vi "Lab Panel V5.10.vi"() -> ()   [LabVIEW 2013] (continued)
                            n1484 = TDMS Write(0:w2790, 5:"TEST PASS", 7:w2794, 9:w2793) -> (15:w2796:errorcluster)  [unwired: 2 in, 3 out]
                            n1485 = local write "data file error"(w2796) -> ()
                          }
                          frame #1 {
                            n1486 = Bundle(cluster=w2797, "STATUS"="T-RISE PASS") -> (w2799:T4)  [unwired: 2 in]
                            n1487 = local write "RESULT LAB05-2"(TRUE) -> ()
                            n1488 = local write "DISP LAB05-2"(w2799) -> ()
                          }
                        }
                      }
                      frame False {
                      }
                    }
                  }
                }
              }
            }
          }
          frame #6 {
            # "end test & close test files"
            n1489 = local read "MAIL SETTINGS"() -> (w2805:T7)
            n1490 = Unbundle(w2805) -> ("OUT SERVER ADDRESS"=w2804:string, "FROM ACCOUNT"=w2803:string)  [unwired: 5 out]
            n1491 = stacked-sequence {
              tunnel: w2815 -> [_ _ _ _ _ _ _ _ _ _]
              tunnel: w2816 -> [_ _ _ _ _ _ _ _ _ _]
              tunnel: w2814 -> [_ _ _ _ _ _ _ _ _ _]
              tunnel: w2813 -> [_ _ _ _ _ _ _ _ _ _]
              tunnel: w2812 -> [_ _ _ _ _ _ _ _ _ _]
              tunnel: w2811 -> [_ _ _ _ _ _ _ _ _ _]
              tunnel: w2810 -> [_ _ _ _ _ _ _ _ _ _]
              tunnel: w2809 -> [_ _ _ _ _ _ _ _ _ _]
              tunnel: w2808 -> [_ _ _ _ _ _ _ _ _ _]
              tunnel: w2807 -> [_ _ _ _ _ _ _ _ _ _]
              tunnel: w2804 -> [w2820 w2872 w2920 w2967 w3014 w3061 w3108 w3155 w3202 w3249]
              tunnel: w2803 -> [w2819 w2871 w2919 w2966 w3013 w3060 w3107 w3154 w3201 w3248]
              tunnel: "Mail Test File To:" -> [w2818 w2870 w2918 w2965 w3012 w3059 w3106 w3153 w3200 w3247]
              tunnel: "Mail Test Fail" -> [w2817 w2869 w2917 w2964 w3011 w3058 w3105 w3152 w3199 w3246]
              frame #0 {
                # "LAB01-1"
                n1492 = local read "DISP LAB01-1"() -> (w2824:T4)
                n1493 = local read "run lab01-1"() -> (w2821:bool)
                n1494 = local read "TDMS LAB01-1"() -> (w2822:refnum<k34>)
                n1495 = Unbundle(w2824) -> ("CYCLE"=w2825:dbl, "STATUS"=w2823:string)  [unwired: 1 out]
                n1496 = case shown="True" w2821 {
                  tunnel: w2825 -> [_ w2831]
                  tunnel: w2824 -> [_ w2833]
                  tunnel: w2823 -> [_ w2830]
                  tunnel: w2822 -> [_ w2832]
                  tunnel: w2820 -> [_ w2829]
                  tunnel: w2819 -> [_ w2828]
                  tunnel: w2818 -> [_ w2827]
                  tunnel: w2817 -> [_ w2826]
                  frame False {
                  }
                  frame True {
                    n1497 = Not Equal?(x=w2830, y="RUN") -> (x != y?=w2834:bool)
                    n1498 = Greater?(x=w2831, y=2.0) -> (0:w2836:bool)
                    n1499 = And(x=w2836, y=w2834) -> (x .and. y?=w2835:bool)
                    n1500 = case shown="True" w2835 {
                      tunnel: w2833 -> [_ w2846]
                      tunnel: w2832 -> [_ w2845]
                      tunnel: w2831 -> [_ w2844]
                      tunnel: w2830 -> [_ w2843]
                      tunnel: w2829 -> [_ w2842]
                      tunnel: w2828 -> [_ w2841]
                      tunnel: w2827 -> [_ w2840]
                      tunnel: w2826 -> [_ w2839]
                      frame False {
                      }
                      frame True {
                        n1501 = stacked-sequence {
                          tunnel: w2846 -> [w2850 _ _]
                          tunnel: w2845 -> [_ w2852 _]
                          tunnel: w2844 -> [_ _ _]
                          tunnel: w2843 -> [_ _ w2858]
                          tunnel: w2842 -> [_ _ w2857]
                          tunnel: w2841 -> [_ _ w2856]
                          tunnel: w2840 -> [_ _ w2855]
                          tunnel: w2839 -> [_ _ w2854]
                          frame #0 {
                            w2847 = FALSE
                            n1502 = local write "mail control"("END") -> ()
                            n1503 = Bundle(cluster=w2850) -> (w2849:T4)  [unwired: 3 in]
                            n1504 = local write "DISP LAB01-1"(w2849) -> ()
                            n1505 = local write "O/I  LAB01-1"(w2847) -> ()
                            n1506 = local write "run lab01-1"(w2847) -> ()
                            n1507 = local write "RUN LAB01-1"(w2847) -> ()
                          }
                          frame #1 {
                            n1508 = TDMS Close(11:w2852) -> (0:w2851:errorcluster)  [unwired: 1 in, 1 out]
                            n1509 = local write "data file error"(w2851) -> ()
                          }
                          frame #2 {
                            n1510 = stacked-sequence {
                              tunnel: "LAB01-1" -> [w2860 w2862 _]
                              tunnel: w2858 -> [_ w2868 _]
                              tunnel: w2857 -> [_ w2867 _]
                              tunnel: w2856 -> [_ w2866 _]
                              tunnel: w2855 -> [_ w2865 _]
                              tunnel: w2854 -> [_ w2864 _]
                              frame #0 {
                                n1511 = call "sub vi - defrag tdms v1.vi"("panel id"=w2860) -> ("error out"=w2859:errorcluster)  [unwired: 10 in]
                                n1512 = local write "data file error"(w2859) -> ()
                              }
                              frame #1 {
                                n1513 = Bundle("STATUS"=w2868, "OUT SERVER ADDRESS"=w2867, "FROM ACCOUNT"=w2866, "Mail Test File To:"=w2865, "Mail Test Fail"=w2864) -> (w2861:T25)  [unwired: 1 in]
                                n1514 = call "Save data file (pass-fail) v5.vi"("Input Cluster"=w2861, "panel id"=w2862) -> ("network file save error"=w2863:errorcluster)  [unwired: 8 in, 1 out]
                                n1515 = local write "data file error"(w2863) -> ()
                              }
                              frame #2 {
                              }
                            }
                          }
                        }
                      }
                    }
                  }
                }
              }
              frame #1 {
                # "LAB01-2"
                n1516 = local read "run lab01-2"() -> (w2873:bool)
                n1517 = case shown="True" w2873 {
                  tunnel: w2872 -> [_ w2877]
                  tunnel: w2871 -> [_ w2876]
                  tunnel: w2870 -> [_ w2875]
                  tunnel: w2869 -> [_ w2874]
                  frame False {
                  }
                  frame True {
                    n1518 = local read "DISP LAB01-2"() -> (w2885:T4)
                    n1519 = local read "TDMS LAB01-2"() -> (w2884:refnum<k34>)
                    n1520 = Unbundle(w2885) -> ("CYCLE"=w2879:dbl, "STATUS"=w2878:string)  [unwired: 1 out]
                    n1521 = Not Equal?(x=w2878, y="RUN") -> (x != y?=w2881:bool)
                    n1522 = Greater?(x=w2879, y=2.0) -> (0:w2882:bool)
                    n1523 = And(x=w2882, y=w2881) -> (x .and. y?=w2880:bool)
                    n1524 = case shown="True" w2880 {
                      tunnel: w2885 -> [_ w2894]
                      tunnel: w2884 -> [_ w2893]
                      tunnel: w2879 -> [_ w2892]
                      tunnel: w2878 -> [_ w2891]
                      tunnel: w2877 -> [_ w2890]
                      tunnel: w2876 -> [_ w2889]
                      tunnel: w2875 -> [_ w2888]
                      tunnel: w2874 -> [_ w2887]
                      frame False {
                      }
                      frame True {
                        n1525 = stacked-sequence {
                          tunnel: w2894 -> [w2897 _ _]
                          tunnel: w2893 -> [_ w2899 _]
                          tunnel: w2892 -> [_ _ _]
                          tunnel: w2891 -> [_ _ w2905]
                          tunnel: w2890 -> [_ _ w2904]
                          tunnel: w2889 -> [_ _ w2903]
                          tunnel: w2888 -> [_ _ w2902]
                          tunnel: w2887 -> [_ _ w2901]
                          frame #0 {
                            w2895 = FALSE
                            n1526 = local write "mail control"("END") -> ()
                            n1527 = Bundle(cluster=w2897) -> (w2898:T4)  [unwired: 3 in]
                            n1528 = local write "RUN LAB01-2"(w2895) -> ()
                            n1529 = local write "run lab01-2"(w2895) -> ()
                            n1530 = local write "O/I  LAB01-2"(w2895) -> ()
                            n1531 = local write "DISP LAB01-2"(w2898) -> ()
                          }
                          frame #1 {
                            n1532 = TDMS Close(11:w2899) -> (0:w2900:errorcluster)  [unwired: 1 in, 1 out]
                            n1533 = local write "data file error"(w2900) -> ()
                          }
                          frame #2 {
                            n1534 = stacked-sequence {
                              tunnel: "LAB01-2" -> [w2908 w2909]
                              tunnel: w2905 -> [_ w2914]
                              tunnel: w2904 -> [_ w2913]
                              tunnel: w2903 -> [_ w2912]
                              tunnel: w2902 -> [_ w2911]
                              tunnel: w2901 -> [_ w2910]
                              frame #0 {
                                n1535 = call "sub vi - defrag tdms v1.vi"("panel id"=w2908) -> ("error out"=w2907:errorcluster)  [unwired: 10 in]
                                n1536 = local write "data file error"(w2907) -> ()
                              }
                              frame #1 {
                                n1537 = Bundle("STATUS"=w2914, "OUT SERVER ADDRESS"=w2913, "FROM ACCOUNT"=w2912, "Mail Test File To:"=w2911, "Mail Test Fail"=w2910) -> (w2916:T25)  [unwired: 1 in]
                                n1538 = call "Save data file (pass-fail) v5.vi"("Input Cluster"=w2916, "panel id"=w2909) -> ("network file save error"=w2915:errorcluster)  [unwired: 8 in, 1 out]
                                n1539 = local write "data file error"(w2915) -> ()
                              }
                            }
                          }
                        }
                      }
                    }
                  }
                }
              }
              frame #2 {
                # "LAB02-1"
                n1540 = local read "run lab02-1"() -> (w2921:bool)
                n1541 = case shown="True" w2921 {
                  tunnel: w2920 -> [_ w2925]
                  tunnel: w2919 -> [_ w2924]
                  tunnel: w2918 -> [_ w2923]
                  tunnel: w2917 -> [_ w2922]
                  frame False {
                  }
                  frame True {
                    n1542 = local read "DISP LAB02-1"() -> (w2933:T4)
                    n1543 = Unbundle(w2933) -> ("CYCLE"=w2929:dbl, "STATUS"=w2926:string)  [unwired: 1 out]
                    n1544 = local read "TDMS LAB02-1"() -> (w2932:refnum<k34>)
                    n1545 = Not Equal?(x=w2926, y="RUN") -> (x != y?=w2928:bool)
                    n1546 = Greater?(x=w2929, y=2.0) -> (0:w2930:bool)
                    n1547 = And(x=w2930, y=w2928) -> (x .and. y?=w2927:bool)
                    n1548 = case shown="True" w2927 {
                      tunnel: w2933 -> [_ w2941]
                      tunnel: w2932 -> [_ w2940]
                      tunnel: w2926 -> [_ w2939]
                      tunnel: w2925 -> [_ w2938]
                      tunnel: w2924 -> [_ w2937]
                      tunnel: w2923 -> [_ w2936]
                      tunnel: w2922 -> [_ w2935]
                      frame False {
                      }
                      frame True {
                        n1549 = stacked-sequence {
                          tunnel: w2941 -> [w2944 _ _]
                          tunnel: w2940 -> [_ w2946 _]
                          tunnel: w2939 -> [_ _ w2952]
                          tunnel: w2938 -> [_ _ w2951]
                          tunnel: w2937 -> [_ _ w2950]
                          tunnel: w2936 -> [_ _ w2949]
                          tunnel: w2935 -> [_ _ w2948]
                          frame #0 {
                            w2942 = FALSE
                            n1550 = local write "mail control"("END") -> ()
                            n1551 = Bundle(cluster=w2944) -> (w2945:T4)  [unwired: 3 in]
                            n1552 = local write "O/I  LAB02-1"(w2942) -> ()
                            n1553 = local write "RUN LAB02-1"(w2942) -> ()
                            n1554 = local write "run lab02-1"(w2942) -> ()
                            n1555 = local write "DISP LAB02-1"(w2945) -> ()
                          }
                          frame #1 {
                            n1556 = TDMS Close(11:w2946) -> (0:w2947:errorcluster)  [unwired: 1 in, 1 out]
                            n1557 = local write "data file error"(w2947) -> ()
                          }
                          frame #2 {
                            n1558 = stacked-sequence {
                              tunnel: "LAB02-1" -> [w2955 w2962]
                              tunnel: w2952 -> [_ w2960]
                              tunnel: w2951 -> [_ w2959]
                              tunnel: w2950 -> [_ w2958]
                              tunnel: w2949 -> [_ w2957]
                              tunnel: w2948 -> [_ w2956]
                              frame #0 {
                                n1559 = call "sub vi - defrag tdms v1.vi"("panel id"=w2955) -> ("error out"=w2954:errorcluster)  [unwired: 10 in]
                                n1560 = local write "data file error"(w2954) -> ()
                              }
                              frame #1 {
                                n1561 = Bundle("STATUS"=w2960, "OUT SERVER ADDRESS"=w2959, "FROM ACCOUNT"=w2958, "Mail Test File To:"=w2957, "Mail Test Fail"=w2956) -> (w2961:T25)  [unwired: 1 in]
                                n1562 = call "Save data file (pass-fail) v5.vi"("Input Cluster"=w2961, "panel id"=w2962) -> ("network file save error"=w2963:errorcluster)  [unwired: 8 in, 1 out]
                                n1563 = local write "data file error"(w2963) -> ()
                              }
                            }
                          }
                        }
                      }
                    }
                  }
                }
              }
              frame #3 {
                # "LAB02-2"
                n1564 = local read "run lab02-2"() -> (w2968:bool)
                n1565 = case shown="True" w2968 {
                  tunnel: w2967 -> [_ w2972]
                  tunnel: w2966 -> [_ w2971]
                  tunnel: w2965 -> [_ w2970]
                  tunnel: w2964 -> [_ w2969]
                  frame False {
                  }
                  frame True {
                    n1566 = local read "DISP LAB02-2"() -> (w2980:T4)
                    n1567 = local read "TDMS LAB02-2"() -> (w2979:refnum<k34>)
                    n1568 = Unbundle(w2980) -> ("CYCLE"=w2976:dbl, "STATUS"=w2973:string)  [unwired: 1 out]
                    n1569 = Not Equal?(x=w2973, y="RUN") -> (x != y?=w2975:bool)
                    n1570 = Greater?(x=w2976, y=2.0) -> (0:w2977:bool)
                    n1571 = And(x=w2977, y=w2975) -> (x .and. y?=w2974:bool)
                    n1572 = case shown="True" w2974 {
                      tunnel: w2980 -> [_ w2988]
                      tunnel: w2979 -> [_ w2987]
                      tunnel: w2973 -> [_ w2986]
                      tunnel: w2972 -> [_ w2985]
                      tunnel: w2971 -> [_ w2984]
                      tunnel: w2970 -> [_ w2983]
                      tunnel: w2969 -> [_ w2982]
                      frame False {
                      }
                      frame True {
                        n1573 = stacked-sequence {
                          tunnel: w2988 -> [w2991 _ _]
                          tunnel: w2987 -> [_ w2993 _]
                          tunnel: w2986 -> [_ _ w2999]
                          tunnel: w2985 -> [_ _ w2998]
                          tunnel: w2984 -> [_ _ w2997]
                          tunnel: w2983 -> [_ _ w2996]
                          tunnel: w2982 -> [_ _ w2995]
                          frame #0 {
                            w2989 = FALSE
                            n1574 = local write "mail control"("END") -> ()
                            n1575 = Bundle(cluster=w2991) -> (w2992:T4)  [unwired: 3 in]
                            n1576 = local write "O/I  LAB02-2"(w2989) -> ()
                            n1577 = local write "run lab02-2"(w2989) -> ()
                            n1578 = local write "RUN LAB02-2"(w2989) -> ()
                            n1579 = local write "DISP LAB02-2"(w2992) -> ()
                          }
                          frame #1 {
                            n1580 = TDMS Close(11:w2993) -> (0:w2994:errorcluster)  [unwired: 1 in, 1 out]
                            n1581 = local write "data file error"(w2994) -> ()
                          }
                          frame #2 {
                            n1582 = stacked-sequence {
                              tunnel: "LAB02-2" -> [w3002 w3008]
                              tunnel: w2999 -> [_ w3007]
                              tunnel: w2998 -> [_ w3006]
                              tunnel: w2997 -> [_ w3005]
                              tunnel: w2996 -> [_ w3004]
                              tunnel: w2995 -> [_ w3003]
                              frame #0 {
                                n1583 = call "sub vi - defrag tdms v1.vi"("panel id"=w3002) -> ("error out"=w3001:errorcluster)  [unwired: 10 in]
                                n1584 = local write "data file error"(w3001) -> ()
                              }
                              frame #1 {
                                n1585 = Bundle("STATUS"=w3007, "OUT SERVER ADDRESS"=w3006, "FROM ACCOUNT"=w3005, "Mail Test File To:"=w3004, "Mail Test Fail"=w3003) -> (w3010:T25)  [unwired: 1 in]
                                n1586 = call "Save data file (pass-fail) v5.vi"("Input Cluster"=w3010, "panel id"=w3008) -> ("network file save error"=w3009:errorcluster)  [unwired: 8 in, 1 out]
                                n1587 = local write "data file error"(w3009) -> ()
                              }
                            }
                          }
                        }
                      }
                    }
                  }
                }
              }
              frame #4 {
                # "LAB03-1"
                n1588 = local read "run lab03-1"() -> (w3015:bool)
                n1589 = case shown="True" w3015 {
                  tunnel: w3014 -> [_ w3019]
                  tunnel: w3013 -> [_ w3018]
                  tunnel: w3012 -> [_ w3017]
                  tunnel: w3011 -> [_ w3016]
                  frame False {
                  }
                  frame True {
                    n1590 = local read "DISP LAB03-1"() -> (w3027:T4)
                    n1591 = local read "TDMS LAB03-1"() -> (w3026:refnum<k34>)
                    n1592 = Unbundle(w3027) -> ("CYCLE"=w3023:dbl, "STATUS"=w3020:string)  [unwired: 1 out]
                    n1593 = Not Equal?(x=w3020, y="RUN") -> (x != y?=w3022:bool)
                    n1594 = Greater?(x=w3023, y=2.0) -> (0:w3024:bool)
                    n1595 = And(x=w3024, y=w3022) -> (x .and. y?=w3021:bool)
                    n1596 = case shown="True" w3021 {
                      tunnel: w3027 -> [_ w3035]
                      tunnel: w3026 -> [_ w3034]
                      tunnel: w3020 -> [_ w3033]
                      tunnel: w3019 -> [_ w3032]
                      tunnel: w3018 -> [_ w3031]
                      tunnel: w3017 -> [_ w3030]
                      tunnel: w3016 -> [_ w3029]
                      frame False {
                      }
                      frame True {
                        n1597 = stacked-sequence {
                          tunnel: w3035 -> [w3038 _ _]
                          tunnel: w3034 -> [_ w3040 _]
                          tunnel: w3033 -> [_ _ w3046]
                          tunnel: w3032 -> [_ _ w3045]
                          tunnel: w3031 -> [_ _ w3044]
                          tunnel: w3030 -> [_ _ w3043]
                          tunnel: w3029 -> [_ _ w3042]
                          frame #0 {
                            w3036 = FALSE
                            n1598 = local write "mail control"("END") -> ()
                            n1599 = Bundle(cluster=w3038) -> (w3039:T4)  [unwired: 3 in]
                            n1600 = local write "O/I  LAB03-1"(w3036) -> ()
                            n1601 = local write "run lab03-1"(w3036) -> ()
                            n1602 = local write "RUN LAB03-1"(w3036) -> ()
                            n1603 = local write "DISP LAB03-1"(w3039) -> ()
                          }
                          frame #1 {
                            n1604 = TDMS Close(11:w3040) -> (0:w3041:errorcluster)  [unwired: 1 in, 1 out]
                            n1605 = local write "data file error"(w3041) -> ()
                          }
                          frame #2 {
                            n1606 = stacked-sequence {
                              tunnel: "LAB03-1" -> [w3049 w3055]
                              tunnel: w3046 -> [_ w3054]
                              tunnel: w3045 -> [_ w3053]
                              tunnel: w3044 -> [_ w3052]
                              tunnel: w3043 -> [_ w3051]
                              tunnel: w3042 -> [_ w3050]
                              frame #0 {
                                n1607 = call "sub vi - defrag tdms v1.vi"("panel id"=w3049) -> ("error out"=w3048:errorcluster)  [unwired: 10 in]
                                n1608 = local write "data file error"(w3048) -> ()
                              }
                              frame #1 {
                                n1609 = Bundle("STATUS"=w3054, "OUT SERVER ADDRESS"=w3053, "FROM ACCOUNT"=w3052, "Mail Test File To:"=w3051, "Mail Test Fail"=w3050) -> (w3057:T25)  [unwired: 1 in]
                                n1610 = call "Save data file (pass-fail) v5.vi"("Input Cluster"=w3057, "panel id"=w3055) -> ("network file save error"=w3056:errorcluster)  [unwired: 8 in, 1 out]
                                n1611 = local write "data file error"(w3056) -> ()
                              }
                            }
                          }
                        }
                      }
                    }
                  }
                }
              }
              frame #5 {
                # "LAB03-2"
                n1612 = local read "run lab03-2"() -> (w3062:bool)
                n1613 = case shown="True" w3062 {
                  tunnel: w3061 -> [_ w3066]
                  tunnel: w3060 -> [_ w3065]
                  tunnel: w3059 -> [_ w3064]
                  tunnel: w3058 -> [_ w3063]
                  frame False {
                  }
                  frame True {
                    n1614 = local read "DISP LAB03-2"() -> (w3074:T4)
                    n1615 = Unbundle(w3074) -> ("CYCLE"=w3070:dbl, "STATUS"=w3067:string)  [unwired: 1 out]
                    n1616 = local read "TDMS LAB03-2"() -> (w3073:refnum<k34>)
                    n1617 = Not Equal?(x=w3067, y="RUN") -> (x != y?=w3069:bool)
                    n1618 = Greater?(x=w3070, y=2.0) -> (0:w3071:bool)
                    n1619 = And(x=w3071, y=w3069) -> (x .and. y?=w3068:bool)
                    n1620 = case shown="True" w3068 {
                      tunnel: w3074 -> [_ w3082]
                      tunnel: w3073 -> [_ w3081]
                      tunnel: w3067 -> [_ w3080]
                      tunnel: w3066 -> [_ w3079]
                      tunnel: w3065 -> [_ w3078]
                      tunnel: w3064 -> [_ w3077]
                      tunnel: w3063 -> [_ w3076]
                      frame False {
                      }
                      frame True {
                        n1621 = stacked-sequence {
                          tunnel: w3082 -> [w3085 _ _]
                          tunnel: w3081 -> [_ w3087 _]
                          tunnel: w3080 -> [_ _ w3093]
                          tunnel: w3079 -> [_ _ w3092]
                          tunnel: w3078 -> [_ _ w3091]
                          tunnel: w3077 -> [_ _ w3090]
                          tunnel: w3076 -> [_ _ w3089]
                          frame #0 {
                            w3083 = FALSE
                            n1622 = local write "mail control"("END") -> ()
                            n1623 = Bundle(cluster=w3085) -> (w3086:T4)  [unwired: 3 in]
                            n1624 = local write "RUN LAB03-2"(w3083) -> ()
                            n1625 = local write "O/I  LAB03-2"(w3083) -> ()
                            n1626 = local write "DISP LAB03-2"(w3086) -> ()
                            n1627 = local write "run lab03-2"(w3083) -> ()
                          }
                          frame #1 {
                            n1628 = TDMS Close(11:w3087) -> (0:w3088:errorcluster)  [unwired: 1 in, 1 out]
                            n1629 = local write "data file error"(w3088) -> ()
                          }
                          frame #2 {
                            n1630 = stacked-sequence {
                              tunnel: "LAB03-2" -> [w3096 w3097]
                              tunnel: w3093 -> [_ w3102]
                              tunnel: w3092 -> [_ w3101]
                              tunnel: w3091 -> [_ w3100]
                              tunnel: w3090 -> [_ w3099]
                              tunnel: w3089 -> [_ w3098]
                              frame #0 {
                                n1631 = call "sub vi - defrag tdms v1.vi"("panel id"=w3096) -> ("error out"=w3095:errorcluster)  [unwired: 10 in]
                                n1632 = local write "data file error"(w3095) -> ()
                              }
                              frame #1 {
                                n1633 = Bundle("STATUS"=w3102, "OUT SERVER ADDRESS"=w3101, "FROM ACCOUNT"=w3100, "Mail Test File To:"=w3099, "Mail Test Fail"=w3098) -> (w3104:T25)  [unwired: 1 in]
                                n1634 = call "Save data file (pass-fail) v5.vi"("Input Cluster"=w3104, "panel id"=w3097) -> ("network file save error"=w3103:errorcluster)  [unwired: 8 in, 1 out]
                                n1635 = local write "data file error"(w3103) -> ()
                              }
                            }
                          }
                        }
                      }
                    }
                  }
                }
              }
              frame #6 {
                # "LAB04-1"
                n1636 = local read "run lab04-1"() -> (w3109:bool)
                n1637 = case shown="True" w3109 {
                  tunnel: w3108 -> [_ w3113]
                  tunnel: w3107 -> [_ w3112]
                  tunnel: w3106 -> [_ w3111]
                  tunnel: w3105 -> [_ w3110]
                  frame False {
                  }
                  frame True {
                    n1638 = local read "DISP LAB04-1"() -> (w3121:T4)
                    n1639 = Unbundle(w3121) -> ("CYCLE"=w3117:dbl, "STATUS"=w3114:string)  [unwired: 1 out]
                    n1640 = local read "TDMS LAB04-1"() -> (w3120:refnum<k34>)
                    n1641 = Not Equal?(x=w3114, y="RUN") -> (x != y?=w3116:bool)
                    n1642 = Greater?(x=w3117, y=2.0) -> (0:w3118:bool)
                    n1643 = And(x=w3118, y=w3116) -> (x .and. y?=w3115:bool)
                    n1644 = case shown="True" w3115 {
                      tunnel: w3121 -> [_ w3129]
                      tunnel: w3120 -> [_ w3128]
                      tunnel: w3114 -> [_ w3127]
                      tunnel: w3113 -> [_ w3126]
                      tunnel: w3112 -> [_ w3125]
                      tunnel: w3111 -> [_ w3124]
                      tunnel: w3110 -> [_ w3123]
                      frame False {
                      }
                      frame True {
                        n1645 = stacked-sequence {
                          tunnel: w3129 -> [w3132 _ _]
                          tunnel: w3128 -> [_ w3134 _]
                          tunnel: w3127 -> [_ _ w3140]
                          tunnel: w3126 -> [_ _ w3139]
                          tunnel: w3125 -> [_ _ w3138]
                          tunnel: w3124 -> [_ _ w3137]
                          tunnel: w3123 -> [_ _ w3136]
                          frame #0 {
                            w3130 = FALSE
                            n1646 = local write "mail control"("END") -> ()
                            n1647 = Bundle(cluster=w3132) -> (w3133:T4)  [unwired: 3 in]
                            n1648 = local write "RUN LAB04-1"(w3130) -> ()
                            n1649 = local write "O/I  LAB04-1"(w3130) -> ()
                            n1650 = local write "run lab04-1"(w3130) -> ()
                            n1651 = local write "DISP LAB04-1"(w3133) -> ()
                          }
                          frame #1 {
                            n1652 = TDMS Close(11:w3134) -> (0:w3135:errorcluster)  [unwired: 1 in, 1 out]
                            n1653 = local write "data file error"(w3135) -> ()
                          }
                          frame #2 {
                            n1654 = stacked-sequence {
                              tunnel: "LAB04-1" -> [w3143 w3144]
                              tunnel: w3140 -> [_ w3149]
                              tunnel: w3139 -> [_ w3148]
                              tunnel: w3138 -> [_ w3147]
                              tunnel: w3137 -> [_ w3146]
                              tunnel: w3136 -> [_ w3145]
                              frame #0 {
                                n1655 = call "sub vi - defrag tdms v1.vi"("panel id"=w3143) -> ("error out"=w3142:errorcluster)  [unwired: 10 in]
                                n1656 = local write "data file error"(w3142) -> ()
                              }
                              frame #1 {
                                n1657 = Bundle("STATUS"=w3149, "OUT SERVER ADDRESS"=w3148, "FROM ACCOUNT"=w3147, "Mail Test File To:"=w3146, "Mail Test Fail"=w3145) -> (w3151:T25)  [unwired: 1 in]
                                n1658 = call "Save data file (pass-fail) v5.vi"("Input Cluster"=w3151, "panel id"=w3144) -> ("network file save error"=w3150:errorcluster)  [unwired: 8 in, 1 out]
                                n1659 = local write "data file error"(w3150) -> ()
                              }
                            }
                          }
                        }
                      }
                    }
                  }
                }
              }
              frame #7 {
                # "LAB04-2"
                n1660 = local read "run lab04-2"() -> (w3156:bool)
                n1661 = case shown="True" w3156 {
                  tunnel: w3155 -> [_ w3160]
                  tunnel: w3154 -> [_ w3159]
                  tunnel: w3153 -> [_ w3158]
                  tunnel: w3152 -> [_ w3157]
                  frame False {
                  }
                  frame True {
                    n1662 = local read "DISP LAB04-2"() -> (w3168:T4)
                    n1663 = Unbundle(w3168) -> ("CYCLE"=w3164:dbl, "STATUS"=w3161:string)  [unwired: 1 out]
                    n1664 = Not Equal?(x=w3161, y="RUN") -> (x != y?=w3163:bool)
                    n1665 = local read "TDMS LAB04-2"() -> (w3167:refnum<k34>)
                    n1666 = Greater?(x=w3164, y=2.0) -> (0:w3165:bool)
                    n1667 = And(x=w3165, y=w3163) -> (x .and. y?=w3162:bool)
                    n1668 = case shown="True" w3162 {
                      tunnel: w3168 -> [_ w3176]
                      tunnel: w3167 -> [_ w3175]
                      tunnel: w3161 -> [_ w3174]
                      tunnel: w3160 -> [_ w3173]
                      tunnel: w3159 -> [_ w3172]
                      tunnel: w3158 -> [_ w3171]
                      tunnel: w3157 -> [_ w3170]
                      frame False {
                      }
                      frame True {
                        n1669 = stacked-sequence {
                          tunnel: w3176 -> [w3179 _ _]
                          tunnel: w3175 -> [_ w3181 _]
                          tunnel: w3174 -> [_ _ w3187]
                          tunnel: w3173 -> [_ _ w3186]
                          tunnel: w3172 -> [_ _ w3185]
                          tunnel: w3171 -> [_ _ w3184]
                          tunnel: w3170 -> [_ _ w3183]
                          frame #0 {
                            w3177 = FALSE
                            n1670 = local write "mail control"("END") -> ()
                            n1671 = Bundle(cluster=w3179) -> (w3180:T4)  [unwired: 3 in]
                            n1672 = local write "O/I  LAB04-2"(w3177) -> ()
                            n1673 = local write "RUN LAB04-2"(w3177) -> ()
                            n1674 = local write "run lab04-2"(w3177) -> ()
                            n1675 = local write "DISP LAB04-2"(w3180) -> ()
                          }
                          frame #1 {
                            n1676 = TDMS Close(11:w3181) -> (0:w3182:errorcluster)  [unwired: 1 in, 1 out]
                            n1677 = local write "data file error"(w3182) -> ()
                          }
                          frame #2 {
                            n1678 = stacked-sequence {
                              tunnel: "LAB04-2" -> [w3190 w3191]
                              tunnel: w3187 -> [_ w3196]
                              tunnel: w3186 -> [_ w3195]
                              tunnel: w3185 -> [_ w3194]
                              tunnel: w3184 -> [_ w3193]
                              tunnel: w3183 -> [_ w3192]
                              frame #0 {
                                n1679 = call "sub vi - defrag tdms v1.vi"("panel id"=w3190) -> ("error out"=w3189:errorcluster)  [unwired: 10 in]
                                n1680 = local write "data file error"(w3189) -> ()
                              }
                              frame #1 {
                                n1681 = Bundle("STATUS"=w3196, "OUT SERVER ADDRESS"=w3195, "FROM ACCOUNT"=w3194, "Mail Test File To:"=w3193, "Mail Test Fail"=w3192) -> (w3198:T25)  [unwired: 1 in]
                                n1682 = call "Save data file (pass-fail) v5.vi"("Input Cluster"=w3198, "panel id"=w3191) -> ("network file save error"=w3197:errorcluster)  [unwired: 8 in, 1 out]
                                n1683 = local write "data file error"(w3197) -> ()
                              }
                            }
                          }
                        }
                      }
                    }
                  }
                }
              }
              frame #8 {
                # "LAB05-1"
                n1684 = local read "run lab05-1"() -> (w3203:bool)
                n1685 = case shown="True" w3203 {
                  tunnel: w3202 -> [_ w3207]
                  tunnel: w3201 -> [_ w3206]
                  tunnel: w3200 -> [_ w3205]
                  tunnel: w3199 -> [_ w3204]
                  frame False {
                  }
                  frame True {
                    n1686 = local read "DISP LAB05-1"() -> (w3215:T4)
                    n1687 = Unbundle(w3215) -> ("CYCLE"=w3211:dbl, "STATUS"=w3208:string)  [unwired: 1 out]
                    n1688 = Not Equal?(x=w3208, y="RUN") -> (x != y?=w3210:bool)
                    n1689 = local read "TDMS LAB05-1"() -> (w3214:refnum<k34>)
                    n1690 = Greater?(x=w3211, y=2.0) -> (0:w3212:bool)
                    n1691 = And(x=w3212, y=w3210) -> (x .and. y?=w3209:bool)
                    n1692 = case shown="True" w3209 {
                      tunnel: w3215 -> [_ w3223]
                      tunnel: w3214 -> [_ w3222]
                      tunnel: w3208 -> [_ w3221]
                      tunnel: w3207 -> [_ w3220]
                      tunnel: w3206 -> [_ w3219]
                      tunnel: w3205 -> [_ w3218]
                      tunnel: w3204 -> [_ w3217]
                      frame False {
                      }
                      frame True {
                        n1693 = stacked-sequence {
                          tunnel: w3223 -> [w3226 _ _]
                          tunnel: w3222 -> [_ w3228 _]
                          tunnel: w3221 -> [_ _ w3234]
                          tunnel: w3220 -> [_ _ w3233]
                          tunnel: w3219 -> [_ _ w3232]
                          tunnel: w3218 -> [_ _ w3231]
                          tunnel: w3217 -> [_ _ w3230]
                          frame #0 {
                            w3224 = FALSE
                            n1694 = local write "mail control"("END") -> ()
                            n1695 = Bundle(cluster=w3226) -> (w3227:T4)  [unwired: 3 in]
                            n1696 = local write "O/I  LAB05-1"(w3224) -> ()
                            n1697 = local write "RUN LAB05-1"(w3224) -> ()
                            n1698 = local write "run lab05-1"(w3224) -> ()
                            n1699 = local write "DISP LAB05-1"(w3227) -> ()
                          }
                          frame #1 {
                            n1700 = TDMS Close(11:w3228) -> (0:w3229:errorcluster)  [unwired: 1 in, 1 out]
                            n1701 = local write "data file error"(w3229) -> ()
                          }
                          frame #2 {
                            n1702 = stacked-sequence {
                              tunnel: "LAB05-1" -> [w3237 w3243]
                              tunnel: w3234 -> [_ w3242]
                              tunnel: w3233 -> [_ w3241]
                              tunnel: w3232 -> [_ w3240]
                              tunnel: w3231 -> [_ w3239]
                              tunnel: w3230 -> [_ w3238]
                              frame #0 {
                                n1703 = call "sub vi - defrag tdms v1.vi"("panel id"=w3237) -> ("error out"=w3236:errorcluster)  [unwired: 10 in]
                                n1704 = local write "data file error"(w3236) -> ()
                              }
                              frame #1 {
                                n1705 = Bundle("STATUS"=w3242, "OUT SERVER ADDRESS"=w3241, "FROM ACCOUNT"=w3240, "Mail Test File To:"=w3239, "Mail Test Fail"=w3238) -> (w3245:T25)  [unwired: 1 in]
                                n1706 = call "Save data file (pass-fail) v5.vi"("Input Cluster"=w3245, "panel id"=w3243) -> ("network file save error"=w3244:errorcluster)  [unwired: 8 in, 1 out]
                                n1707 = local write "data file error"(w3244) -> ()
                              }
                            }
                          }
                        }
                      }
                    }
                  }
                }
              }
              frame #9 {
                # "LAB05-2"
                n1708 = local read "run lab05-2"() -> (w3250:bool)
                n1709 = case shown="True" w3250 {
                  tunnel: w3249 -> [_ w3254]
                  tunnel: w3248 -> [_ w3253]
                  tunnel: w3247 -> [_ w3252]
                  tunnel: w3246 -> [_ w3251]
                  frame False {
                  }
                  frame True {
                    n1710 = local read "DISP LAB05-2"() -> (w3262:T4)
                    n1711 = Unbundle(w3262) -> ("CYCLE"=w3258:dbl, "STATUS"=w3255:string)  [unwired: 1 out]
                    n1712 = Not Equal?(x=w3255, y="RUN") -> (x != y?=w3257:bool)
                    n1713 = local read "TDMS LAB05-2"() -> (w3261:refnum<k34>)
                    n1714 = Greater?(x=w3258, y=2.0) -> (0:w3259:bool)
                    n1715 = And(x=w3259, y=w3257) -> (x .and. y?=w3256:bool)
                    n1716 = case shown="True" w3256 {
                      tunnel: w3262 -> [_ w3270]
                      tunnel: w3261 -> [_ w3269]
                      tunnel: w3255 -> [_ w3268]
                      tunnel: w3254 -> [_ w3267]
                      tunnel: w3253 -> [_ w3266]
                      tunnel: w3252 -> [_ w3265]
                      tunnel: w3251 -> [_ w3264]
                      frame False {
                      }
                      frame True {
                        n1717 = stacked-sequence {
                          tunnel: w3270 -> [w3273 _ _]
                          tunnel: w3269 -> [_ w3275 _]
                          tunnel: w3268 -> [_ _ w3281]
                          tunnel: w3267 -> [_ _ w3280]
                          tunnel: w3266 -> [_ _ w3279]
                          tunnel: w3265 -> [_ _ w3278]
                          tunnel: w3264 -> [_ _ w3277]
                          frame #0 {
                            w3271 = FALSE
                            n1718 = local write "mail control"("END") -> ()
                            n1719 = Bundle(cluster=w3273) -> (w3274:T4)  [unwired: 3 in]
                            n1720 = local write "RUN LAB05-2"(w3271) -> ()
                            n1721 = local write "O/I  LAB05-2"(w3271) -> ()
                            n1722 = local write "run lab05-2"(w3271) -> ()
                            n1723 = local write "DISP LAB05-2"(w3274) -> ()
                          }
                          frame #1 {
                            n1724 = TDMS Close(11:w3275) -> (0:w3276:errorcluster)  [unwired: 1 in, 1 out]
                            n1725 = local write "data file error"(w3276) -> ()
                          }
                          frame #2 {
                            n1726 = stacked-sequence {
                              tunnel: "LAB05-2" -> [w3284 w3290]
                              tunnel: w3281 -> [_ w3289]
                              tunnel: w3280 -> [_ w3288]
                              tunnel: w3279 -> [_ w3287]
                              tunnel: w3278 -> [_ w3286]
                              tunnel: w3277 -> [_ w3285]
                              frame #0 {
                                n1727 = call "sub vi - defrag tdms v1.vi"("panel id"=w3284) -> ("error out"=w3283:errorcluster)  [unwired: 10 in]
                                n1728 = local write "data file error"(w3283) -> ()
                              }
                              frame #1 {
                                n1729 = Bundle("STATUS"=w3289, "OUT SERVER ADDRESS"=w3288, "FROM ACCOUNT"=w3287, "Mail Test File To:"=w3286, "Mail Test Fail"=w3285) -> (w3292:T25)  [unwired: 1 in]
                                n1730 = call "Save data file (pass-fail) v5.vi"("Input Cluster"=w3292, "panel id"=w3290) -> ("network file save error"=w3291:errorcluster)  [unwired: 8 in, 1 out]
                                n1731 = local write "data file error"(w3291) -> ()
                              }
                            }
                          }
                        }
                      }
                    }
                  }
                }
              }
            }
            n1732 = local read "Network Directory"() -> (w2806:path)
            n1733 = global write "Global 1.vi" "Network Drive"(w2806) -> ()
          }
          frame #7 {
            # "disable functions"
            n1734 = stacked-sequence {
              tunnel: w3302 -> [w3316 _ w3373]
              tunnel: w3301 -> [w3311 _ w3372]
              tunnel: w3300 -> [w3310 _ w3371]
              tunnel: w3299 -> [w3308 _ w3370]
              tunnel: w3298 -> [w3309 _ w3369]
              tunnel: w3297 -> [_ w3333 w3368]
              tunnel: w3296 -> [_ w3334 w3367]
              tunnel: w3295 -> [_ w3335 w3366]
              tunnel: w3294 -> [_ w3336 w3365]
              tunnel: w3293 -> [_ w3337 w3364]
              frame #0 {
                n1735 = Select(t=2, s=w3308, f=0) -> (s? t:f=w3304:i32)
                n1736 = Select(t=2, s=w3310, f=0) -> (s? t:f=w3305:i32)
                n1737 = Select(t=2, s=w3309, f=0) -> (s? t:f=w3303:i32)
                n1738 = Select(t=2, s=w3316, f=0) -> (s? t:f=w3307:i32)
                n1739 = Select(t=2, s=w3311, f=0) -> (s? t:f=w3306:i32)
                n1740 = property on="SELECT LAB02-2" class="RadioBtnsControl (strict)"("DisabledEnum"=w3304) -> ()  [unwired: 2 in, 2 out]
                n1741 = property on="SELECT LAB02-1" class="RadioBtnsControl (strict)"("DisabledEnum"=w3305) -> ()  [unwired: 2 in, 2 out]
                n1742 = property on="SELECT LAB03-1" class="RadioBtnsControl (strict)"("DisabledEnum"=w3303) -> ()  [unwired: 2 in, 2 out]
                n1743 = property on="SELECT LAB01-1" class="RadioBtnsControl (strict)"("DisabledEnum"=w3307) -> ()  [unwired: 2 in, 2 out]
                n1744 = property on="SELECT LAB01-2" class="RadioBtnsControl (strict)"("DisabledEnum"=w3306) -> ()  [unwired: 2 in, 2 out]
                n1745 = Not(x=w3316) -> (.not. x?=w3317:bool)
                n1746 = property on="RESULT LAB01-1" class="Bool (strict)"("Visible"=w3317) -> ()  [unwired: 2 in, 2 out]
                n1747 = Not(x=w3311) -> (.not. x?=w3315:bool)
                n1748 = Not(x=w3310) -> (.not. x?=w3314:bool)
                n1749 = Not(x=w3308) -> (.not. x?=w3313:bool)
                n1750 = property on="RESULT LAB01-2" class="Bool (strict)"("Visible"=w3315) -> ()  [unwired: 2 in, 2 out]
                n1751 = Not(x=w3309) -> (.not. x?=w3312:bool)
                n1752 = property on="RESULT LAB02-1" class="Bool (strict)"("Visible"=w3314) -> ()  [unwired: 2 in, 2 out]
                n1753 = property on="RESULT LAB02-2" class="Bool (strict)"("Visible"=w3313) -> ()  [unwired: 2 in, 2 out]
                n1754 = property on="RESULT LAB03-1" class="Bool (strict)"("Visible"=w3312) -> ()  [unwired: 2 in, 2 out]
                n1755 = property on="SET LAB01-1" class="Clust (strict)"("DisabledEnum"=w3307) -> ()  [unwired: 2 in, 2 out]
                n1756 = property on="SET LAB01-2" class="Clust (strict)"("DisabledEnum"=w3306) -> ()  [unwired: 2 in, 2 out]
                n1757 = property on="SET LAB02-1" class="Clust (strict)"("DisabledEnum"=w3305) -> ()  [unwired: 2 in, 2 out]
                n1758 = property on="SET LAB02-2" class="Clust (strict)"("DisabledEnum"=w3304) -> ()  [unwired: 2 in, 2 out]
                n1759 = property on="SET LAB03-1" class="Clust (strict)"("DisabledEnum"=w3303) -> ()  [unwired: 2 in, 2 out]
                n1760 = property on="O/I  LAB01-1" class="Bool (strict)"("DisabledEnum"=w3307) -> ()  [unwired: 2 in, 2 out]
                n1761 = property on="O/I  LAB01-2" class="Bool (strict)"("DisabledEnum"=w3306) -> ()  [unwired: 2 in, 2 out]
                n1762 = property on="O/I  LAB02-1" class="Bool (strict)"("DisabledEnum"=w3305) -> ()  [unwired: 2 in, 2 out]
                n1763 = property on="O/I  LAB02-2" class="Bool (strict)"("DisabledEnum"=w3304) -> ()  [unwired: 2 in, 2 out]
                n1764 = property on="O/I  LAB03-1" class="Bool (strict)"("DisabledEnum"=w3303) -> ()  [unwired: 2 in, 2 out]
              }
              frame #1 {
                n1765 = Select(t=2, s=w3337, f=0) -> (s? t:f=w3328:i32)
                n1766 = Select(t=2, s=w3336, f=0) -> (s? t:f=w3329:i32)
                n1767 = Select(t=2, s=w3333, f=0) -> (s? t:f=w3332:i32)
                n1768 = Select(t=2, s=w3334, f=0) -> (s? t:f=w3331:i32)
                n1769 = Select(t=2, s=w3335, f=0) -> (s? t:f=w3330:i32)
                n1770 = property on="SELECT LAB05-2" class="RadioBtnsControl (strict)"("DisabledEnum"=w3328) -> ()  [unwired: 2 in, 2 out]
                n1771 = property on="SELECT LAB05-1" class="RadioBtnsControl (strict)"("DisabledEnum"=w3329) -> ()  [unwired: 2 in, 2 out]
                n1772 = property on="SELECT LAB03-2" class="RadioBtnsControl (strict)"("DisabledEnum"=w3332) -> ()  [unwired: 2 in, 2 out]
                n1773 = property on="SELECT LAB04-1" class="RadioBtnsControl (strict)"("DisabledEnum"=w3331) -> ()  [unwired: 2 in, 2 out]
                n1774 = property on="SELECT LAB04-2" class="RadioBtnsControl (strict)"("DisabledEnum"=w3330) -> ()  [unwired: 2 in, 2 out]
                n1775 = property on="SET LAB05-2" class="Clust (strict)"("DisabledEnum"=w3328) -> ()  [unwired: 2 in, 2 out]
                n1776 = property on="SET LAB05-1" class="Clust (strict)"("DisabledEnum"=w3329) -> ()  [unwired: 2 in, 2 out]
                n1777 = property on="SET LAB03-2" class="Clust (strict)"("DisabledEnum"=w3332) -> ()  [unwired: 2 in, 2 out]
                n1778 = property on="SET LAB04-1" class="Clust (strict)"("DisabledEnum"=w3331) -> ()  [unwired: 2 in, 2 out]
                n1779 = property on="SET LAB04-2" class="Clust (strict)"("DisabledEnum"=w3330) -> ()  [unwired: 2 in, 2 out]
